vi "VI Tree.vi"   [LabVIEW 2012, in "MGC647C.lvlib"]
doc: "This is the instrument driver for the <b>MKS 647C</b>. The VI Tree displays all the user-callable VIs of the instrument driver in an organized table."
uses:
  <instrlib>/MGC647C/MGC647C.lvlib
panel:
  # "(C) Copyright 2012 GSI Helmholtzzentrum für Schwerionenforschung GmbH.  ALL RIGHTS RESERVED."
  # "SEE DIAGRAM\nFOR VI TREE."
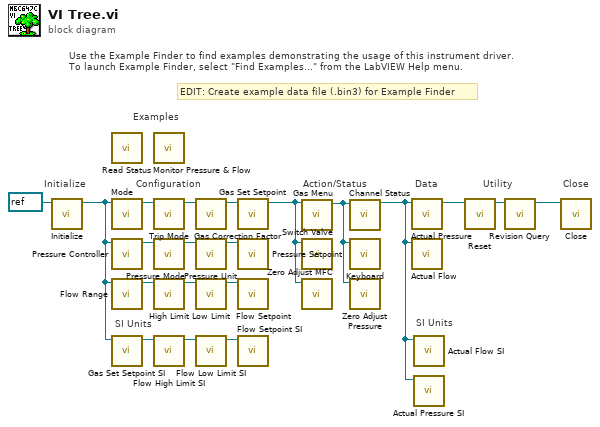
[diagram p0: block diagram]
diagram:
  # "Examples"
  # "SI Units"
  # "SI Units"
  # "EDIT: Create example data file (.bin3) for Example Finder"
  # "Use the Example Finder to find examples demonstrating the usage of this instrument driver.\nTo launch Example Finder, select \"Find Examples...\" from the LabVIEW Help menu."
  # "Configuration"
  # "Utility"
  # "Data"
  # "Action/Status"
  # "Close"
  # "Initialize"
  n1 = call <instrlib>:"Initialize.vi"("VISA resource name"=refnum<visa-resource-name> refnum) -> ("VISA resource name out"=w6:refnum<visa-resource-name>)  [unwired: 9 in, 1 out]
  n2 = call <instrlib>:"Read Status.vi"() -> ()  [unwired: 12 in]
  n3 = call <instrlib>:"Mode.vi"("VISA resource name"=w6) -> ("dup VISA resource name"=w12:refnum<visa-resource-name>)  [unwired: 7 in, 3 out]
  n4 = call <instrlib>:"Pressure Controller.vi"("VISA resource name"=w6) -> ("dup VISA resource name"=w13:refnum<visa-resource-name>)  [unwired: 8 in, 2 out]
  n5 = call <instrlib>:"Flow Range.vi"("VISA resource name"=w6) -> ("dup VISA resource name"=w9:refnum<visa-resource-name>)  [unwired: 8 in, 2 out]
  n6 = call <instrlib>:"Gas Set Setpoint SI.vi"("VISA resource name"=w6) -> ("dup VISA resource name"=w5:refnum<visa-resource-name>)  [unwired: 8 in, 2 out]
  n7 = call <instrlib>:"Monitor Pressure & Flow.vi"() -> ()  [unwired: 12 in]
  n8 = call <instrlib>:"Trip Mode.vi"("VISA resource name"=w12) -> ("dup VISA resource name"=w11:refnum<visa-resource-name>)  [unwired: 8 in, 2 out]
  n9 = call <instrlib>:"Pressure Mode.vi"("VISA resource name"=w13) -> ("dup VISA resource name"=w15:refnum<visa-resource-name>)  [unwired: 8 in, 2 out]
  n10 = call <instrlib>:"High Limit.vi"("VISA resource name"=w9) -> ("dup VISA resource name"=w8:refnum<visa-resource-name>)  [unwired: 8 in, 2 out]
  n11 = call <instrlib>:"Flow High Limit SI.vi"("VISA resource name"=w5) -> ("dup VISA resource name"=w4:refnum<visa-resource-name>)  [unwired: 8 in, 2 out]
  n12 = call <instrlib>:"Gas Correction Factor.vi"("VISA resource name"=w11) -> ("dup VISA resource name"=w10:refnum<visa-resource-name>)  [unwired: 8 in, 2 out]
  n13 = call <instrlib>:"Pressure Unit.vi"("VISA resource name"=w15) -> ("dup VISA resource name"=w14:refnum<visa-resource-name>)  [unwired: 8 in, 2 out]
  n14 = call <instrlib>:"Low Limit.vi"("VISA resource name"=w8) -> ("dup VISA resource name"=w7:refnum<visa-resource-name>)  [unwired: 8 in, 2 out]
  n15 = call <instrlib>:"Flow Low Limit SI.vi"("VISA resource name"=w4) -> ("dup VISA resource name"=w3:refnum<visa-resource-name>)  [unwired: 8 in, 2 out]
  n16 = call <instrlib>:"Gas Set Setpoint.vi"("VISA resource name"=w10) -> ("dup VISA resource name"=w2:refnum<visa-resource-name>)  [unwired: 8 in, 2 out]
  n17 = call <instrlib>:"Pressure Setpoint.vi"("VISA resource name"=w14) -> ()  [unwired: 8 in, 3 out]
  n18 = call <instrlib>:"Flow Setpoint.vi"("VISA resource name"=w7) -> ()  [unwired: 8 in, 3 out]
  n19 = call <instrlib>:"Flow Setpoint SI.vi"("VISA resource name"=w3) -> ()  [unwired: 8 in, 3 out]
  n20 = call <instrlib>:"Gas Menu.vi"("VISA resource name"=w2) -> ("dup VISA resource name"=w16:refnum<visa-resource-name>)  [unwired: 8 in, 2 out]
  n21 = call <instrlib>:"Switch Valve.vi"("VISA resource name"=w2) -> ()  [unwired: 9 in, 2 out]
  n22 = call <instrlib>:"Zero Adjust MFC.vi"("VISA resource name"=w2) -> ()  [unwired: 8 in, 3 out]
  n23 = call <instrlib>:"Channel Status.vi"("VISA resource name"=w16) -> ("dup VISA resource name"=w1:refnum<visa-resource-name>)  [unwired: 7 in, 3 out]
  n24 = call <instrlib>:"Keyboard.vi"("VISA resource name"=w16) -> ()  [unwired: 9 in, 2 out]
  n25 = call <instrlib>:"Zero Adjust Pressure.vi"("VISA resource name"=w16) -> ()  [unwired: 8 in, 3 out]
  n26 = call <instrlib>:"Actual Pressure.vi"("VISA resource name"=w1) -> ("dup VISA resource name"=w17:refnum<visa-resource-name>)  [unwired: 8 in, 2 out]
  n27 = call <instrlib>:"Actual Flow.vi"("VISA resource name"=w1) -> ()  [unwired: 8 in, 3 out]
  n28 = call <instrlib>:"Actual Flow SI.vi"("VISA resource name"=w1) -> ()  [unwired: 8 in, 3 out]
  n29 = call <instrlib>:"Actual Pressure SI.vi"("VISA resource name"=w1) -> ()  [unwired: 8 in, 3 out]
  n30 = call <instrlib>:"Reset.vi"("VISA resource name"=w17) -> ("VISA resource name out"=w19:refnum<visa-resource-name>)  [unwired: 9 in, 1 out]
  n31 = call <instrlib>:"Revision Query.vi"("VISA resource name"=w19) -> ("VISA resource name out"=w18:refnum<visa-resource-name>)  [unwired: 7 in, 3 out]
  n32 = call <instrlib>:"Close.vi"("VISA resource name"=w18) -> ()  [unwired: 10 in, 1 out]
